vi "AlliGator Save Multiple Phasor Plots Additional Data.vi"(4 "Save only if selected":bool, 6 "Save as...":bool, 7 "Phasor Plot Path (empty)":path, 8 "error in (no error)":errorcluster, 9 "Raw Phasor Plots":T1[](array[typedef]) {"[Decay Metadata]"."# Folds" min=1; "[Decay Metadata]"."ROI Descriptor"."Contours"."Type" items=["No Selection", "Point", "Line", "Rectangle", "Oval", "Polygon", "Freehand Region", "Annulus", "Unused2", "Unused3", "Broken Line", "Freehand Line", "Rotated Rectangle"]}, 10 "All Plots":bool, 11 "Phasor Graph":refnum<vi>) -> (0 "Error Out":errorcluster, 1 "Message":string)   [LabVIEW 2021, in "AlliGator Phasor Graph.lvlib"]
doc: "Save phasor plot additional data to an ASCII file."
uses:
  AlliGator Phasor Graph.lvlib
  AlliGator Raw Phasor Plot Data v4.ctl
  Phasor/Phasor (g, s).ctl
  AlliGator Decay Metadata v3.ctl
  Decay Analysis/Decay Preprocessing/AlliGator Decay Background Subtraction Info.ctl
  Decay Analysis/Decay Preprocessing/AlliGator Baseline Subtraction Method.ctl
  Graphs/XY Graph/XY Graph Plot Shift Parameters.ctl
  Graphs/XY Graph/XY Graph Plot Shift Method.ctl
  Decay Analysis/Decay Preprocessing/AlliGator Decay Extrapolation Parameters.ctl
  Phasor/Phasor Standard Deviation Options.ctl
  Phasor/Calibration Phasor (m, phi).ctl
  Graphs/XY Graph/XY Graph Add-Ons.lvlib
  Strings/Strings.lvlib
  Phasor/Phasor.lvlib
  Decay Analysis/Decay Preprocessing/AlliGator Decay Preprocessing.lvlib
panel:
  # "see the AlliGator License on the block diagram (Ctrl+E or Window:Show Block Diagram)"
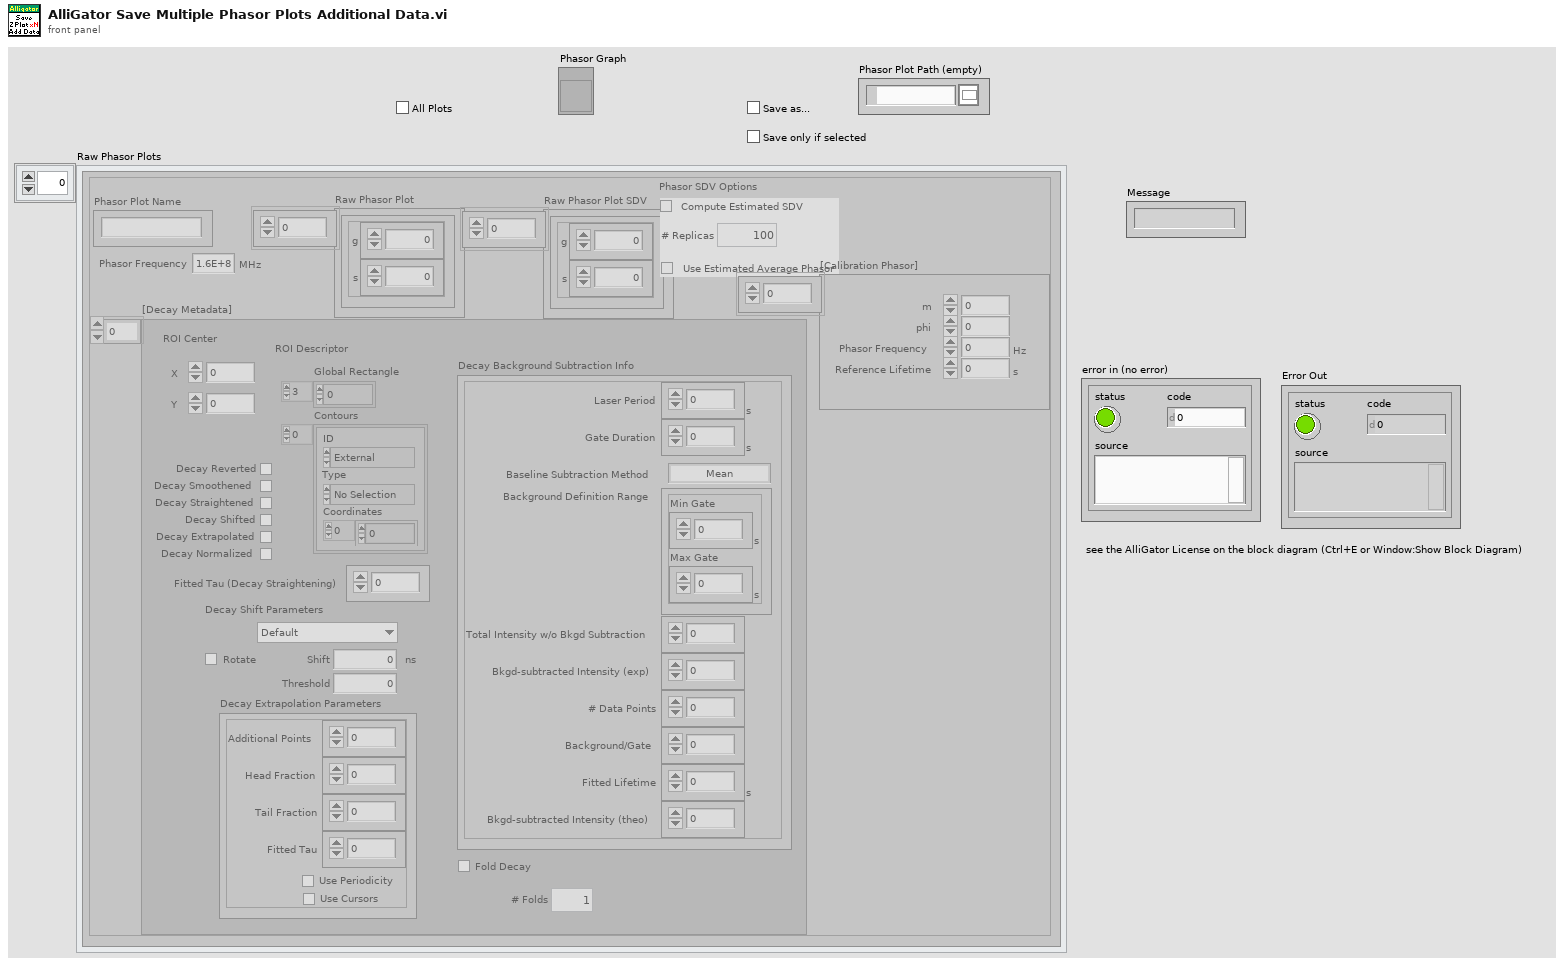
[diagram p1: front panel]
types:
  T1 = typedef "AlliGator Phasor Graph.lvlib/AlliGator Raw Phasor Plot Data v4.ctl" = cluster{"Phasor Plot Name":string, "Raw Phasor Plot":T2[], "Phasor Frequency":dbl[unit], "[Decay Metadata]":T3[], "Raw Phasor Plot SDV":T2[], "Phasor SDV Options":T10, "[Calibration Phasor]":T11[]}
  T2 = typedef "Phasor.lvlib/Phasor (g, s).ctl" = cluster{"g":dbl, "s":dbl}
  T3 = typedef "AlliGator Phasor Graph.lvlib/AlliGator Decay Metadata v3.ctl" = cluster{"ROI Descriptor":T4, "ROI Center":cluster{"X":i32, "Y":i32}, "Decay Background Subtraction Info":T5, "Decay Reverted":bool, "Decay Smoothened":bool, "Decay Straightened":bool, "Fitted Tau (Decay Straightening)":dbl, "Decay Shift Parameters":T7, "Decay Shifted":bool, "Decay Extrapolated":bool, "Decay Extrapolation Parameters":T9, "Decay Normalized":bool, "Fold Decay":bool, "# Folds":u32}
  T4 = typedef "ROI Descriptor" = cluster{"Global Rectangle":i32[], "Contours":cluster{"ID":enum32{"External", "Internal"}, "Type":u32, "Coordinates":i32[]}[]}
  T5 = typedef "AlliGator Decay Preprocessing.lvlib/AlliGator Decay Background Subtraction Info.ctl" = cluster{"Laser Period":dbl[unit], "Gate Duration":dbl[unit], "Baseline Subtraction Method":T6, "Background Definition Range":cluster{"Min Gate":dbl[unit], "Max Gate":dbl[unit]}, "Total Intensity w/o Bkgd Subtraction":dbl, "Bkgd-subtracted Intensity (exp)":dbl, "# Data Points":i32, "Background/Gate":dbl, "Fitted Lifetime":dbl[unit], "Bkgd-subtracted Intensity (theo)":dbl}
  T6 = typedef "AlliGator Decay Preprocessing.lvlib/AlliGator Baseline Subtraction Method.ctl" = enum16{"Mean", "Min", "Square Gated Single-Exponential", "File", "Constant"}
  T7 = typedef "XY Graph Add-Ons.lvlib/XY Graph Plot Shift Parameters.ctl" = cluster{"Type":T8, "Shift":dbl[unit], "Threshold":dbl, "Rotate":bool}
  T8 = typedef "XY Graph Add-Ons.lvlib/XY Graph Plot Shift Method.ctl" = enum16{"Default", "CFD", "Threshold", "Cross-Correlation"}
  T9 = typedef "AlliGator Decay Preprocessing.lvlib/AlliGator Decay Extrapolation Parameters.ctl" = cluster{"Additional Points":u32, "Head Fraction":dbl, "Fitted Tau":dbl, "Use Periodicity":bool, "Use Cursors":bool, "Tail Fraction":dbl}
  T10 = typedef "Phasor.lvlib/Phasor Standard Deviation Options.ctl" = cluster{"Compute Estimated SDV":bool, "# Replicas":u32, "Use Estimated Average Phasor":bool}
  T11 = typedef "Phasor.lvlib/Calibration Phasor (m, phi).ctl" = cluster{"m":dbl, "phi":dbl, "Phasor Frequency":dbl[unit], "Reference Lifetime":dbl[unit]}
  T12 = typedef "XY Graph Add-Ons.lvlib/XY Graph Refnum.ctl" = refnum<vi>
  T13 = typedef "AlliGator Phasor Graph.lvlib/AlliGator Phasor Plot Exported Data Selection.ctl" = cluster{"x":bool, "y":bool, "g":bool, "s":bool, "phi":bool, "m":bool, "tau phi":bool, "tau m":bool, "phasor ratio (intensity-weighted)":bool, "<tau> (intensity-weighted)":bool, "phasor ratio (amplitude-weighted)":bool, "<tau> (amplitude-weighted)":bool, "g SDV":bool, "s SDV":bool, "phi SDV":bool, "m SDV":bool, "tau phi SDV":bool, "tau m SDV":bool, "phasor ratio (intensity-weighted) SDV":bool, "<tau> (intensity-weighted) SDV":bool, "phasor ratio (amplitude-weighted) SDV":bool, "<tau> (amplitude-weighted) SDV":bool}
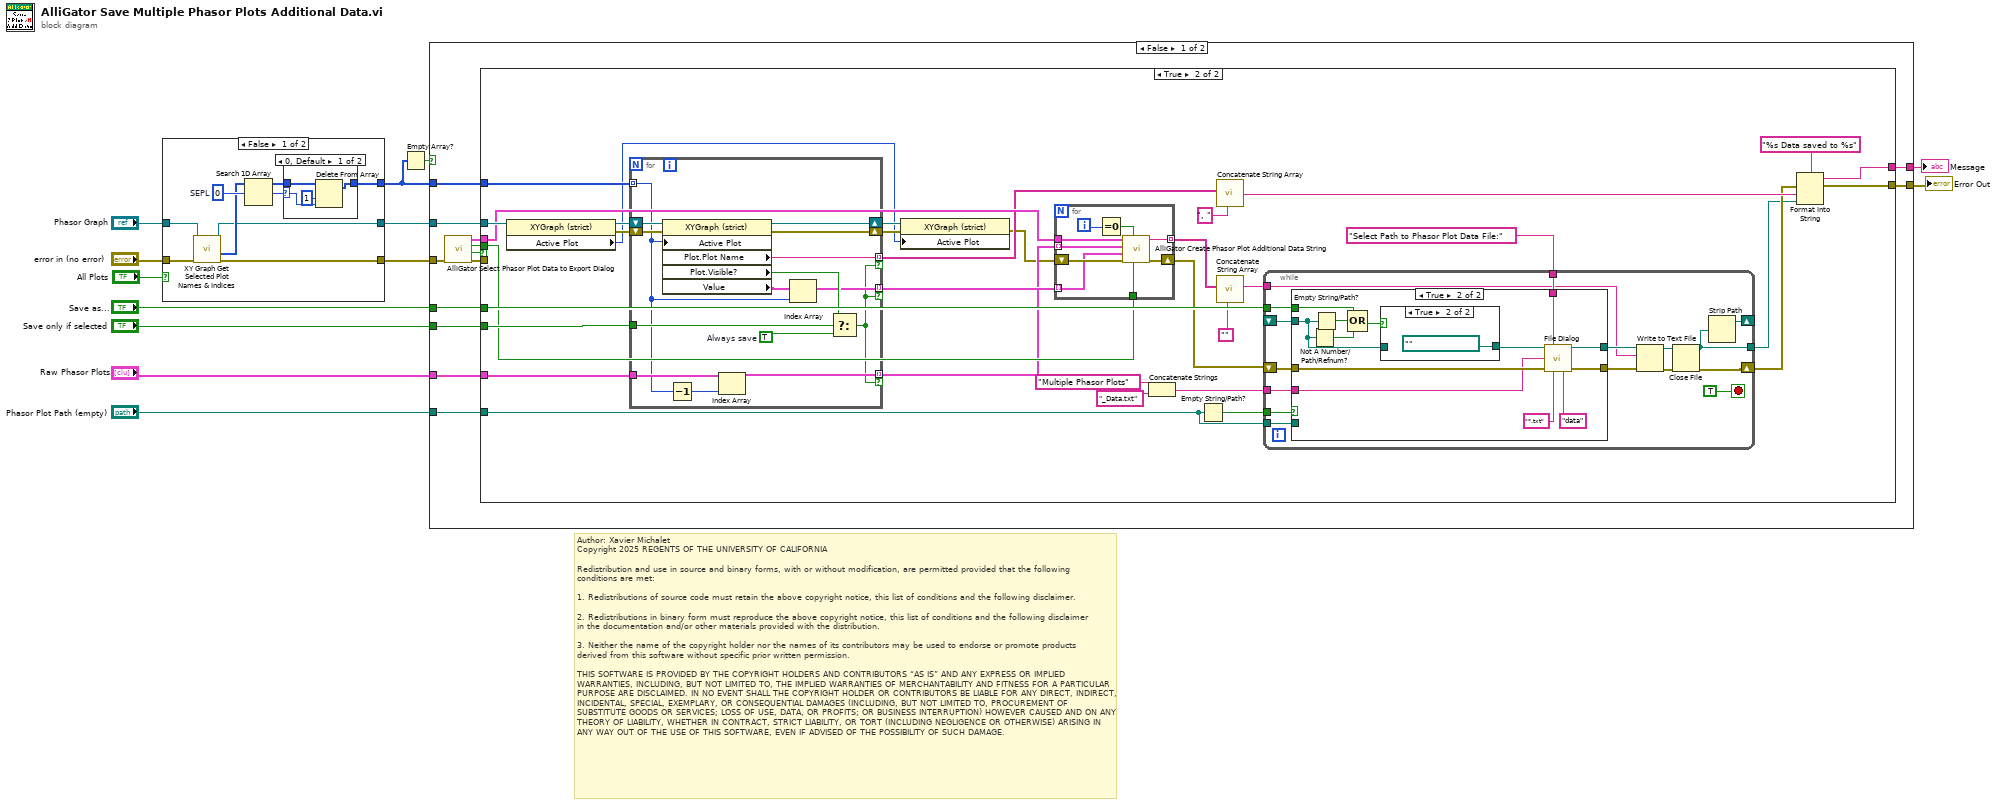
[diagram p0: block diagram]
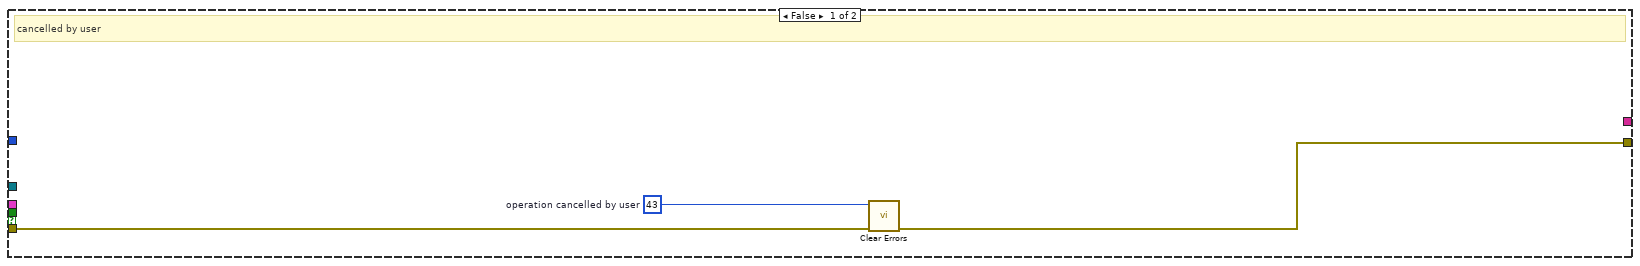
[diagram p2: hidden frame]
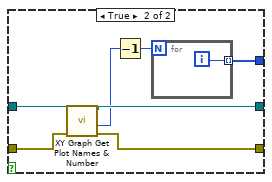
[diagram p7: hidden frame]
diagram:
  # "Author: Xavier Michalet\nCopyright 2025 REGENTS OF THE UNIVERSITY OF CALIFORNIA\n\nRedistribution and use in source and binary forms, with or without modification, are permitted provided that the following conditions are met:\n\n1. Redistributions of source code must retain the above copyright notice, this list of conditions and the following disclaimer.\n\n2. Redistributions in binary form must reproduce the above copyright notice, this list of conditions and the following disclaimer in the documentation and/or other materials provided with the distribution.\n\n3. Neither the name of the copyright holder nor the names of its contributors may be used to endorse or promote products derived from this software without specific prior written permission.\n\nTHIS SOFTWARE IS PROVIDED BY THE COPYRIGHT HOLDERS AND CONTRIBUTORS “AS IS” AND ANY EXPRESS OR IMPLIED WARRANTIES, INCLUDING, BUT NOT LIMITED TO, THE IMPLIED WARRANTIES OF MERCHANTABILITY AND FITNESS FOR A PARTICULAR PURPOSE ARE DISCLAIMED. IN NO EVENT SHALL THE COPYRIGHT HOLDER OR CONTRIBUTORS BE LIABLE FOR ANY DIRECT, INDIRECT, INCIDENTAL, SPECIAL, EXEMPLARY, OR CONSEQUENTIAL DAMAGES (INCLUDING, BUT NOT LIMITED TO, PROCUREMENT OF SUBSTITUTE GOODS OR SERVICES; LOSS OF USE, DATA, OR PROFITS; OR BUSINESS INTERRUPTION) HOWEVER CAUSED AND ON ANY THEORY OF LIABILITY, WHETHER IN CONTRACT, STRICT LIABILITY, OR TORT (INCLUDING NEGLIGENCE OR OTHERWISE) ARISING IN ANY WAY OUT OF THE USE OF THIS SOFTWARE, EVEN IF ADVISED OF THE POSSIBILITY OF SUCH DAMAGE."
  n1 = case shown="False" "All Plots" {
    tunnel: "error in (no error)" -> [w21 w32]
    tunnel: [w20 w30] -> w7
    tunnel: "Phasor Graph" -> [w16 w33]
    tunnel: [w15 w31] -> w5
    tunnel: [w14 w27] -> w3
    frame False {
      w19 = 0  # SEPL
      n2 = call "XY Graph Get Selected Plot Names & Indices.vi"("error in (no error)"=w21, "XYGraph in"=w16) -> ("error out"=w20:errorcluster, "Selected Plots"=w17:i32[], "XYGraph out"=w15:T12)  [unwired: 5 in, 2 out]
      n3 = Search 1D Array(1D array=w17, element=w19) -> (index of element=w18:i32)  [unwired: 1 in]
      n4 = case shown="0, Default" w18 {
        selector: w18 -> [w22 _]
        tunnel: w17 -> [w25 w26]
        tunnel: [w24 w26] -> w14
        frame 0, Default {
          n5 = Delete From Array(array=w25, length=1, index=w22) -> (array with subset deleted=w24:i32[])  [unwired: 1 out]
        }
        frame -1 {
        }
      }
    }
    frame True {
      n6 = call "XY Graph Get Plot Names & Number.vi"("error in (no error)"=w32, "XYGraph in"=w33) -> ("error out"=w30:errorcluster, "# Plots"=w29:i32, "XYGraph out"=w31:T12)  [unwired: 4 in, 3 out]
      n7 = Decrement(x=w29) -> (x-1=w28:i32)
      n8 = for {
        N: w28 -> [_]
        tunnel: [w34] -> w27 mode=indexing
        i -> [w34]
      }
    }
  }
  n9 = Empty Array?(array=w3) -> (empty?=w4:bool)
  n10 = case shown="False" w4 {
    tunnel: [w47 w141] -> w13
    tunnel: "Raw Phasor Plots" -> [w46 _]
    tunnel: "Save as..." -> [w45 _]
    tunnel: "Phasor Plot Path (empty)" -> [w44 _]
    tunnel: "Save only if selected" -> [w43 _]
    tunnel: w7 -> [w38 w141]
    tunnel: w5 -> [w37 _]
    tunnel: w3 -> [w36 _]
    tunnel: [w35 _] -> w1
    frame False {
      n11 = call "AlliGator Select Phasor Plot Data to Export Dialog.vi"("error in (no error)"=w38) -> ("error out"=w42:errorcluster, "OK?"=w41:bool, "Average Plot Data"=w39:bool, "Phasor Plot Exported Data"=w40:T13)  [unwired: 7 in]
      n12 = case shown="True" w41 {
        tunnel: w37 -> [_ w83]
        tunnel: [w49 w51] -> w47
        tunnel: w46 -> [_ w63]
        tunnel: w45 -> [_ w78]
        tunnel: w44 -> [_ w76]
        tunnel: w43 -> [_ w75]
        tunnel: w42 -> [w50 _]
        tunnel: w40 -> [_ w74]
        tunnel: w39 -> [_ w73]
        tunnel: w36 -> [_ w65]
        tunnel: [_ w52] -> w35
        frame False {
          w48 = 43  # operation cancelled by user
          # "cancelled by user"
          n13 = call <vilib>:"Clear Errors.vi"("error in (no error)"=w50, "specific error code to clear (0: all)"=w48) -> ("error out"=w49:errorcluster)  [unwired: 4 in, 1 out]
        }
        frame True {
          n14 = property class="XYGraph (strict)"(reference=w83) -> (reference out=w82:T12, error out=w81:errorcluster, "Active Plot"=w58:u32)  [unwired: 1 in]
          n15 = for {
            tunnel: [w131] -> w68 mode=indexing if=w126
            shift-right: [w135] -> w60
            shift-left: w81 -> [w139]
            tunnel: w75 -> [w138]
            shift-right: [w133] -> w61
            shift-left: w82 -> [w140]
            tunnel: w65 -> [w129] mode=indexing
            tunnel: [w132] -> w64 mode=indexing if=w126
            tunnel: w63 -> [w130]
            tunnel: [w127] -> w62 mode=indexing if=w126
            w137 = TRUE  # Always save
            n16 = property class="XYGraph (strict)"(reference=w140, error in=w139, "Active Plot"=w129) -> (reference out=w133:T12, error out=w135:errorcluster, "Plot.Plot Name"=w132:string, "Plot.Visible?"=w136:bool, "Value"=w134:cluster{"X Array":dbl[], "Y Array":dbl[]}[])
            n17 = Decrement(x=w129) -> (x-1=w128:i32)
            n18 = Index Array(array=w130, index=w128) -> (element=w127:T1)
            n19 = Index Array(array=w134, index=w129) -> (element=w131:cluster{"X Array":dbl[], "Y Array":dbl[]})
            n20 = Select(t=w136, s=w138, f=w137) -> (s? t:f=w126:bool)
          }
          n21 = property class="XYGraph (strict)"(reference=w61, error in=w60, "Active Plot"=w58) -> (error out=w59:errorcluster)  [unwired: 1 out]
          n22 = for {
            tunnel: [w125] -> w70 mode=indexing
            tunnel: w74 -> [w124]
            tunnel: w62 -> [w122] mode=indexing
            tunnel: w73 -> [w121]
            shift-right: [w120] -> w72
            shift-left: w59 -> [w123]
            tunnel: w68 -> [w117] mode=indexing
            i -> [w119]
            n23 = Equal To 0?(x=w119) -> (x = 0?=w118:bool)
            n24 = call "AlliGator Create Phasor Plot Additional Data String.vi"("Average Plot Data (F)"=w121, "Include Header String (F)"=w118, "error in (no error)"=w123, "Calibrated Phasor Plot"=w117, "Raw Phasor Plot"=w122, "Phasor Plot Exported Data"=w124) -> ("error out"=w120:errorcluster, "Phasor Plot Additional Data String"=w125:string)  [unwired: 4 in]
          }
          n25 = Concatenate Strings("Multiple Phasor Plots" ("string"), "_Data.txt" ("string")) -> (w79:string)
          n26 = Empty String/Path?(string/path=w76) -> (empty?=w77:bool)
          n27 = call "Concatenate String Array.vi"("Separator (TAB)"=", ", "String Array"=w64) -> ("Formatted String"=w66:string)  [unwired: 9 in]
          n28 = call "Concatenate String Array.vi"("Separator (TAB)"="", "String Array"=w70) -> ("Formatted String"=w69:string)  [unwired: 9 in]
          n29 = while {
            tunnel: w69 -> [w90]
            tunnel: [w86] -> w55
            shift-right: [w87] -> w56
            shift-left: w72 -> [w94]
            shift-right: [w99] -> _
            shift-left: _ -> [w96]
            tunnel: w78 -> [w97]
            tunnel: "Select Path to Phasor Plot Data File:" ("Prompt") -> [w95]
            tunnel: w79 -> [w93]
            tunnel: w77 -> [w85]
            tunnel: w76 -> [w84]
            stop <- TRUE stop-if-true
            n30 = case shown="True" w85 {
              tunnel: w97 -> [_ w112]
              tunnel: w96 -> [_ w110]
              tunnel: w95 -> [_ w108]
              tunnel: w94 -> [w100 w107]
              tunnel: w93 -> [_ w104]
              tunnel: [w101 w103] -> w92
              tunnel: [w100 w102] -> w91
              tunnel: w84 -> [w101 _]
              frame False {
              }
              frame True {
                n31 = Not A Number/Path/Refnum?(number/path/refnum=w110) -> (NaN/Path/Refnum?=w113:bool)
                n32 = Empty String/Path?(string/path=w110) -> (empty?=w114:bool)
                n33 = Compound Arithmetic op=OR(w112, w114, w113) -> (w111:bool)
                n34 = case shown="True" w111 {
                  tunnel: [w115 path "" ("start path  (Not A Path)")] -> w109
                  tunnel: w110 -> [w115 _]
                  frame False {
                  }
                  frame True {
                  }
                }
                n35 = call "File Dialog"("start path"=w109, "prompt"=w108, "default name"=w104, "error in"=w107, "pattern (all files)"="*.txt" ("Pattern (*.xml;*.XML)"), "pattern label"="data" ("File Extension (xml)")) -> ("selected path"=w103:path, "error out"=w102:errorcluster)  [unwired: 6 in, 2 out]
              }
            }
            n36 = Write to Text File(file (use dialog)=w92, text=w90, error in=w91) -> (refnum out=w89:refnum<file>, error out=w88:errorcluster)  [unwired: 1 in, 1 out]
            n37 = Close File(refnum=w89, error in=w88) -> (path=w86:path, error out=w87:errorcluster)
            n38 = Strip Path(path=w86) -> (stripped path=w99:path)  [unwired: 1 out]
          }
          n39 = Format Into String(format string="%s Data saved to %s", error in=w56, w66, w55) -> (resulting string=w52:string, error out=w51:errorcluster)  [unwired: 1 in]
        }
      }
    }
    frame True {
      # "No valid selected plot"
    }
  }
  "Error Out" <- w13
  "Message" <- w1
